vi "Call_back.vi"(4 "ContexMenue":refnum<class "ContexMenue.lvclass">, 5 "Event Data":cluster{"sender":refnum<k24>, "e":refnum<k24>}, 6 "Control Ref":refnum<k24>, 7 "Event Common Data":T1) -> ()   [LabVIEW 2016, in "NotifyIcon.lvclass"]
uses:
  NotifyIcon.lvclass
  System.Windows.Forms
  ContexMenue/ContexMenue.lvclass
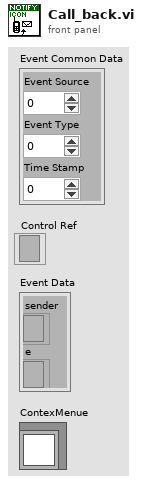
[diagram p1: front panel]
types:
  T1 = cluster{"Event Source":i32, "Event Type":u32, "Time Stamp":u32}
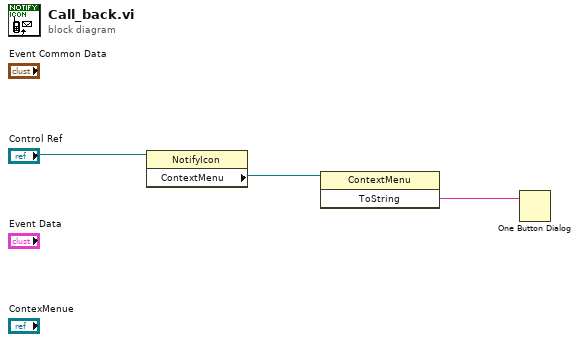
[diagram p0: block diagram]
diagram:
  n1 = property class="NotifyIcon"(reference="Control Ref") -> ("ContextMenu"=w2:refnum<k24>)  [unwired: 1 in, 2 out]
  n2 = invoke class="ContextMenu" method="ToString"(reference=w2) -> ("ToString"=w1:string)  [unwired: 2 in, 2 out]
  n3 = One Button Dialog(message=w1) -> ()  [unwired: 1 in, 1 out]
